vi "IMUrollpitch.vi"(5 "v(m/s)":dbl, 7 "SteeringAngle(rad/s)":dbl, 8 "PrevRoll(deg)":dbl, 9 "Bias":T2, 10 "PrevFilteredGyro(deg)":T1, 11 "error in (no error)":errorcluster) -> (0 "Roll(deg)":dbl, 2 "FilteredGyro(deg)":T1, 3 "error out":errorcluster)   [LabVIEW 2016]
doc: "Inputs\nPrevious roll (deg)\nPrevious filtered gyro values (deg)\nIMU Bias\nForward velocity (m/s)\nSteering angle (rad)\n\nOutput\nCurrent Roll angle (deg)\nCurrent filtred gyro readings (deg)\n\n\n\nCalculates the roll angle using gyro and accelerometer values and neglects the bias values from the measurements. The equations are based from documentation from chalmers."
uses:
  <vilib>/imath/engines/lvmath2/RunTimeEngine/BuiltInFunctions/atan2/NIMS_atan2.vi
  <instcachedir>/0/NIMS_atan2_A91AA4A7D42247EDBE8F76DB99AF04A4.lvgen/NIMS_atan2_A91AA4A7D42247EDBE8F76DB99AF04A4_000.vi
  <vilib>/imath/engines/lvmath2/RunTimeEngine/NodeEndStatement/NIMS_NodeEndStatement_Output.vi
  <instcachedir>/0/NIMS_NodeEndStatement_Output_53EC0D466D134D7ABD903AC30B43404B.lvgen/NIMS_NodeEndStatement_Output_53EC0D466D134D7ABD903AC30B43404B_001.vi
  <vilib>/imath/engines/lvmath2/RunTimeEngine/ErrorHandling/NIMS_Finalize Error.vi
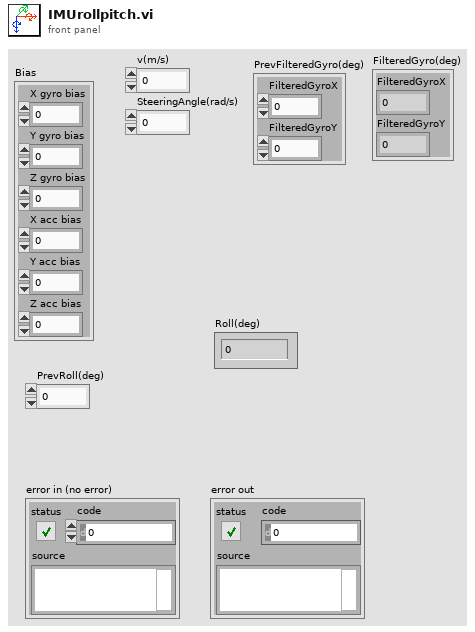
[diagram p1: front panel]
types:
  T1 = cluster{"FilteredGyroX":dbl, "FilteredGyroY":dbl}
  T2 = cluster{"X gyro bias":dbl, "Y gyro bias":dbl, "Z gyro bias":dbl, "X acc bias":dbl, "Y acc bias":dbl, "Z acc bias":dbl}
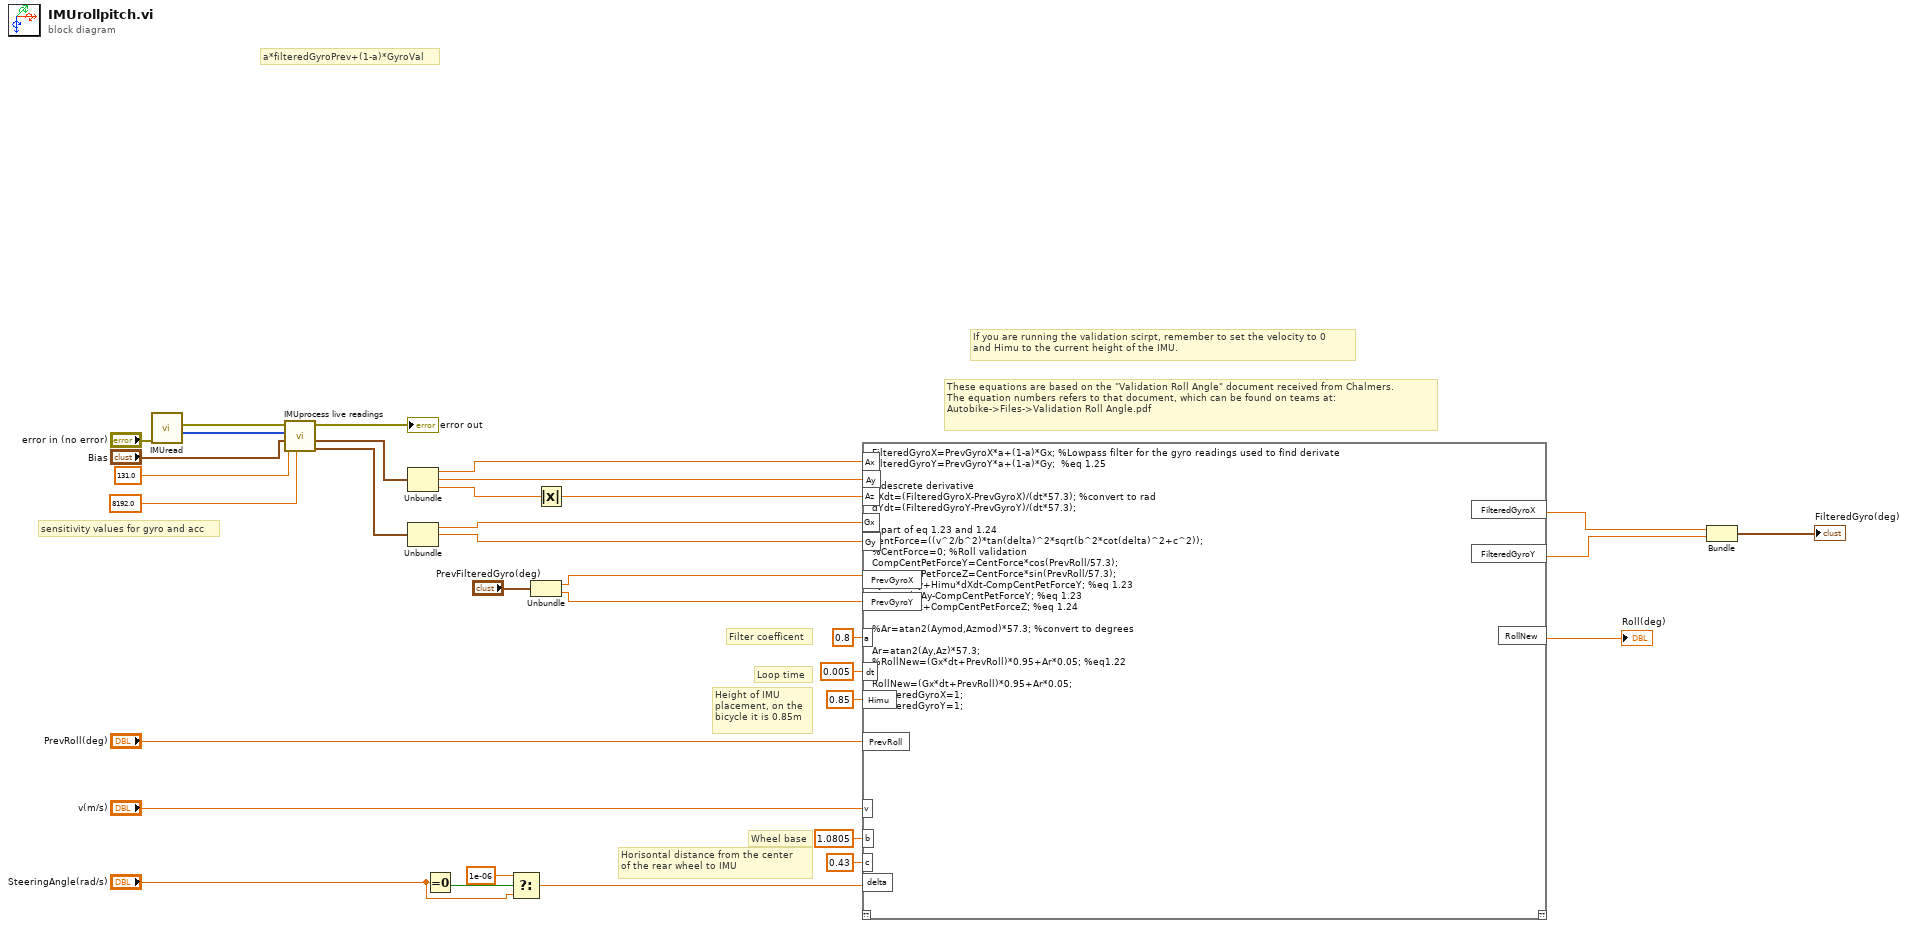
[diagram p0: block diagram]
diagram:
  # "Horisontal distance from the center \nof the rear wheel to IMU"
  # "Filter coefficent"
  # "Wheel base"
  # "These equations are based on the \"Validation Roll Angle\" document received from Chalmers.\nThe equation numbers refers to that document, which can be found on teams at:\nAutobike->Files->Validation Roll Angle.pdf"
  # "If you are running the validation scirpt, remember to set the velocity to 0\nand Himu to the current height of the IMU."
  # "sensitivity values for gyro and acc"
  # "Loop time"
  # "Height of IMU\nplacement, on the\nbicycle it is 0.85m"
  # "a*filteredGyroPrev+(1-a)*GyroVal"
  n1 = call "IMUread.vi"("error in (no error)"="error in (no error)") -> ("error out"=w29:errorcluster, "Accel, Gyro"=w27:u16[])  [unwired: 9 in]
  n2 = call "IMUprocess live readings.vi"("Acc sensivity"=8192.0 ("Acc s"), "Gyro sensivity"=131.0 ("Gyro s"), "Bias"="Bias", "Sensor Data in"=w27, "error in (no error)"=w29) -> ("Gyro deg/s"=w19:cluster{dbl, dbl, dbl}, "Accel g's"=w20:cluster{dbl, dbl, dbl}, "error out"=→"error out":errorcluster)  [unwired: 4 in]
  n3 = Unbundle(w20) -> (w22:dbl, w3:dbl, w1:dbl)
  n4 = Unbundle(w19) -> (w4:dbl, w5:dbl)  [unwired: 1 out]
  n5 = Equal To 0?(x="SteeringAngle(rad/s)") -> (x = 0?=w15:bool)
  n6 = Select(t=1e-06, s=w15, f="SteeringAngle(rad/s)") -> (s? t:f=w13:dbl)
  n7 = Unbundle("PrevFilteredGyro(deg)") -> ("FilteredGyroX"=w7:dbl, "FilteredGyroY"=w6:dbl)
  n8 = Absolute Value(x=w1) -> (abs(x)=w2:dbl)
  n9 = mathscript code="FilteredGyroX=PrevGyroX*a+(1-a)*Gx; %Lowpass filter for the gyro readings used to find derivate\nFilteredGyroY=PrevGyroY*a+(1-a)*Gy;  %eq 1.25\n\n%descrete derivative\ndXdt=(FilteredGyroX-PrevGyroX)/(dt*57.3); %convert to rad\ndYdt=(FilteredGyroY-PrevGyroY)/(dt*57.3); \n\n%part of eq 1.23 and 1.24\nCentForce=((v^2/b^2)*tan(delta)^2*sqrt(b^2*cot(delta)^2+c^2));\n%CentForce=0; %Roll validation\nCompCentPetForceY=CentForce*cos(PrevRoll/57.3);\nCompCentPetForceZ=CentForce*sin(PrevRoll/57.3);\nAymod=Ay+Himu*dXdt-CompCentPetForceY; %eq 1.23 \n%Aymod=Ay-CompCentPetForceY; %eq 1.23 \nAzmod=Az+CompCentPetForceZ; %eq 1.24\n\n%Ar=atan2(Aymod,Azmod)*57.3; %convert to degrees\n\nAr=atan2(Ay,Az)*57.3;\n%RollNew=(Gx*dt+PrevRoll)*0.95+Ar*0.05; %eq1.22\n\nRollNew=(Gx*dt+PrevRoll)*0.95+Ar*0.05;\n%FilteredGyroX=1;\n%FilteredGyroY=1;"("Ax"=w22, "Ay"=w3, "Az"=w2, "Gx"=w4, "Gy"=w5, "PrevRoll"="PrevRoll(deg)", "PrevGyroX"=w7, "PrevGyroY"=w6, "a"=0.8, "dt"=0.005, "Himu"=0.85, "v"="v(m/s)", "b"=1.0805, "c"=0.43, "delta"=w13) -> ("RollNew"=→"Roll(deg)":dbl, "FilteredGyroX"=w11:dbl, "FilteredGyroY"=w10:dbl)  [unwired: 1 in, 1 out]
  n10 = Bundle("FilteredGyroX"=w11, "FilteredGyroY"=w10) -> (→"FilteredGyro(deg)":T1)  [unwired: 1 in]
